vi "RichToFlatcif_plugincore_TimingStatsBasic.vi"(5 "OutputClusterType":T1, 11 "InputCluster":T2) -> (3 "OutputCluster":T1)   [LabVIEW 2021, in "CIFCorePlugin_client.lvlib"]
uses:
  CIFCorePlugin_client.lvlib
  cif_plugincore_TimingStatsBasic.ctl
  cif_plugincore_TimingStatsBasic_Flat.ctl
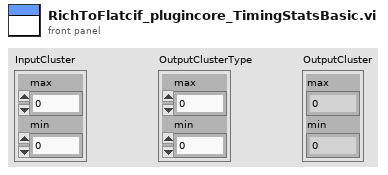
[diagram p1: front panel]
types:
  T1 = typedef "CIFCorePlugin_client.lvlib/cif_plugincore_TimingStatsBasic_Flat.ctl" = cluster{"max":i32, "min":i32}
  T2 = typedef "CIFCorePlugin_client.lvlib/cif_plugincore_TimingStatsBasic.ctl" = cluster{"max":i32, "min":i32}
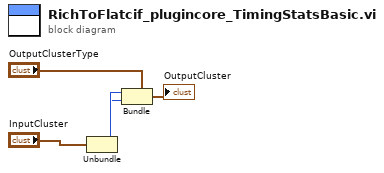
[diagram p0: block diagram]
diagram:
  n1 = Unbundle "Unbundle"("InputCluster") -> ("max"=w2:i32, "min"=w1:i32)
  n2 = Bundle "Bundle"(cluster="OutputClusterType", "max"=w2, "min"=w1) -> (→"OutputCluster":T1)
